vi "Ex2.vi"() -> ()   [LabVIEW 2016]
panel:
  out "클릭 횟수":i32
  in  "정지":bool
  out "LED":bool
  in  "스위치":bool
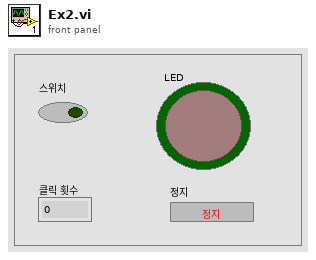
[diagram p1: front panel]
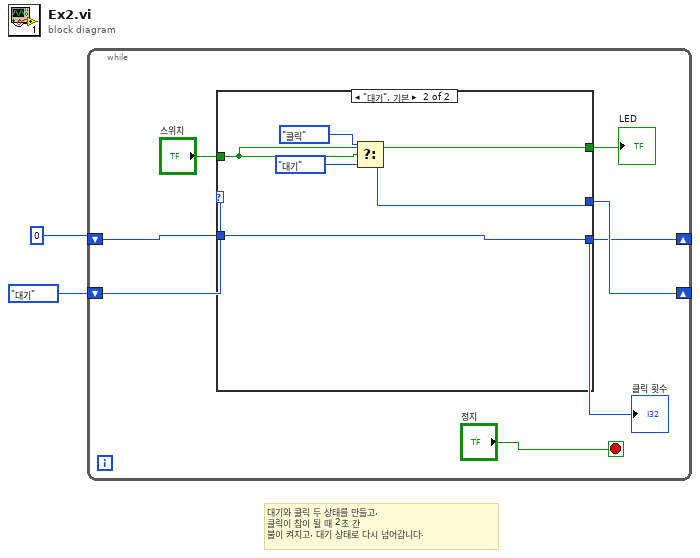
[diagram p0: block diagram]
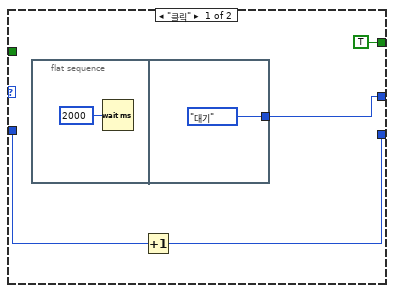
[diagram p2: hidden frame]
diagram:
  # "대기와 클릭 두 상태를 만들고, \n클릭이 참이 될 때 2초 간 \n불이 켜지고, 대기 상태로 다시 넘어갑니다."
  n1 = while {
    shift-right: [w4] -> _
    shift-left: 0 -> [w7]
    shift-right: [w5] -> _
    shift-left: enum16{"클릭", "대기"}."대기" -> [w8]
    stop <- "정지" stop-if-true
    n2 = case shown="\"대기\", 기본" w8 {
      tunnel: w7 -> [w12 w20]
      tunnel: [w13 w20] -> w4
      tunnel: "스위치" -> [_ w16]
      tunnel: [w10 w19] -> w5
      tunnel: [TRUE ("불리언") w16] -> w3
      frame "클릭" {
        n3 = flat-sequence {
          tunnel: [enum16{"클릭", "대기"}."대기"] -> w10
          frame #0 {
            n4 = Wait (ms)(milliseconds to wait=u32 2000 ("대기 시간 (ms)")) -> ()  [unwired: 1 out]
          }
          frame #1 {
          }
        }
        n5 = Increment(x=w12) -> (x+1=w13:i32)
      }
      frame "대기", Default {
        n6 = Select(t=enum16{"클릭", "대기"}."클릭", s=w16, f=enum16{"클릭", "대기"}."대기") -> (s? t:f=w19:enum16{"클릭", "대기"})
      }
    }
    "LED" <- w3
    "클릭 횟수" <- w4
  }
